vi "CloseLogFile.vi"(0 "Buffers in":T1={"Channels"=[], "PosttriggerBuffer"=refnum, "PretriggerBuffer"=refnum, "BlockSizePerChannel"=0, " logging semaphore"=refnum, "Log refnum"=refnum, "snapshotBuffer"=refnum, "logDirectory"=path "", "logPrefix"="", "decimation factor"=1, "max files"=0, "SampleRate"=0.0}, 11 "error in (no error)":errorcluster) -> (4 "Buffers out":T1={"Channels"=[], "PosttriggerBuffer"=refnum, "PretriggerBuffer"=refnum, "BlockSizePerChannel"=0, " logging semaphore"=refnum, "Log refnum"=refnum, "snapshotBuffer"=refnum, "logDirectory"=path "", "logPrefix"="", "decimation factor"=1, "max files"=0, "SampleRate"=0.0}, 6 "log path out":path, 15 "error out":errorcluster)   [LabVIEW 2017, in "BufferLogging.lvlib"]
uses:
  BufferLogging.lvlib
  Buffers.ctl
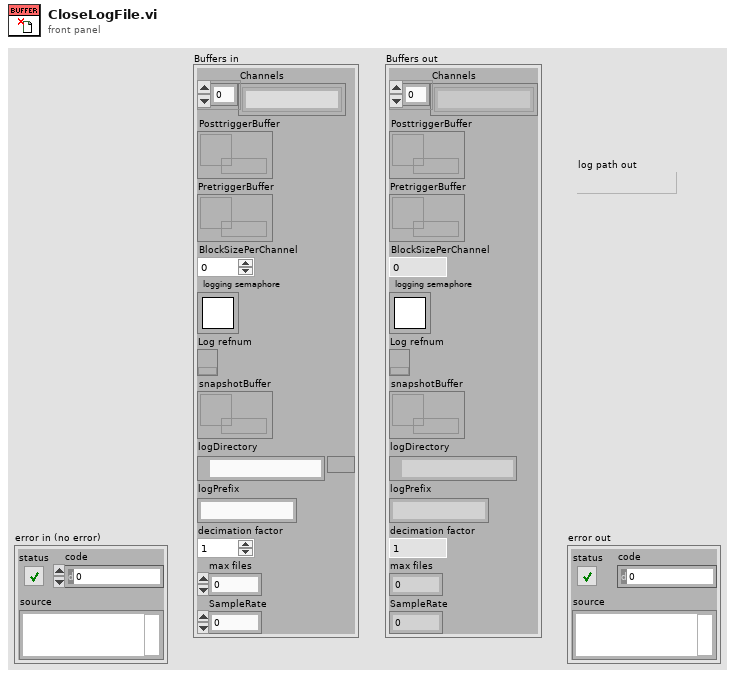
[diagram p1: front panel]
types:
  T1 = typedef "BufferLogging.lvlib/Buffers.ctl" = cluster{"Channels":string[], "PosttriggerBuffer":refnum<queue>, "PretriggerBuffer":refnum<queue>, "BlockSizePerChannel":i32, " logging semaphore":T2, "Log refnum":refnum<k34>, "snapshotBuffer":refnum<data-value>, "logDirectory":path, "logPrefix":string, "decimation factor":i32, "max files":i32, "SampleRate":dbl}
  T2 = typedef "Semaphore RefNum" = refnum<k1>
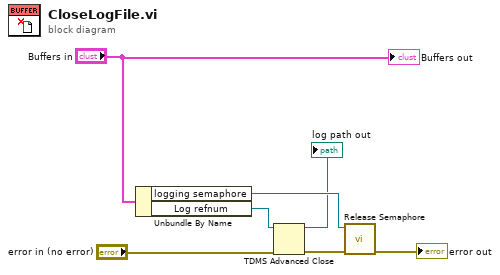
[diagram p0: block diagram]
diagram:
  n1 = Unbundle By Name("Buffers in") -> ("logging semaphore"=w3:T2, "Log refnum"=w6:refnum<k34>)
  n2 = TDMS Advanced Close(8:"error in (no error)", 11:w6) -> (0:w5:errorcluster, 3:→"log path out":path)  [unwired: 2 in]
  n3 = call <vilib>:"Release Semaphore.vi"("error in (no error)"=w5, "semaphore"=w3) -> ("error out"=→"error out":errorcluster)  [unwired: 4 in, 1 out]
  "Buffers out" <- "Buffers in"
